vi "Tag Conflict Error Message.vi"(6 "Previous Error Message":string, 8 "error in (no error)":errorcluster, 9 "Tag Name":string, 10 "Conflict Class":string, 11 "Original Class":string) -> (0 "error out":errorcluster, 4 "Error Message":string)   [LabVIEW 2021, in "Var Bus.lvclass"]
uses:
  Var Bus.lvclass
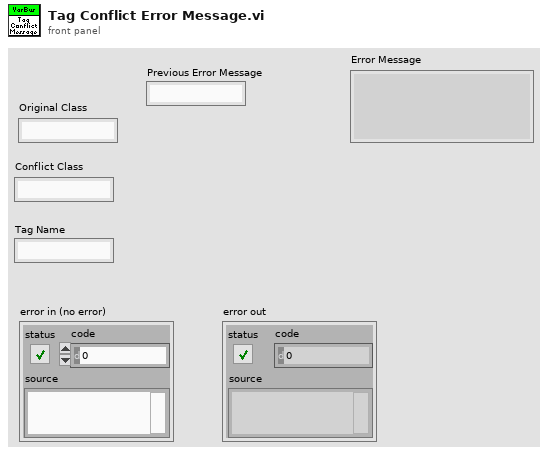
[diagram p1: front panel]
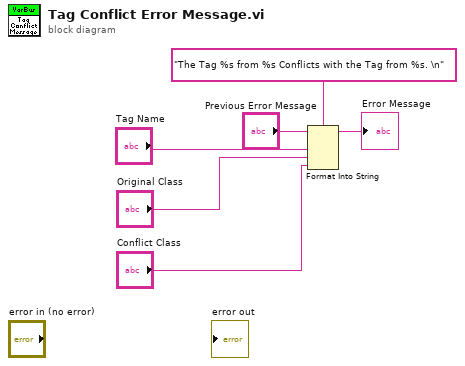
[diagram p0: block diagram]
diagram:
  n1 = Format Into String(format string="The Tag %s from %s Conflicts with the Tag from %s. \n", initial string="Previous Error Message", "Tag Name", "Original Class", "Conflict Class") -> (resulting string=→"Error Message":string)  [unwired: 1 in, 1 out]
